vi "S4GUI_001.vi"() -> ()   [LabVIEW 2018] (continued)
            n2478 = call-dynamic "Read State Machine.vi"("error in (no error)"=w5934, "Device in"=w5935) -> ("error out"=w5938:errorcluster, "State Machine.lvclass"=w5931:refnum<class "State Machine.lvclass">, "Device out"=w5933:refnum<class "Channel.lvclass">)  [unwired: 7 in]
            n2479 = call "Next State.vi"("error in (no error)"=w5938, "New_State"=12, "State Machine in"=w5931) -> ("error out"=w5937:errorcluster, "State Machine out"=w5930:refnum<class "State Machine.lvclass">)  [unwired: 7 in]
            n2480 = call-dynamic "Write State Machine.vi"("error in (no error)"=w5937, "State Machine.lvclass"=w5930, "Device in"=w5933) -> ("error out"=w5929:errorcluster, "Device out"=w5932:refnum<class "Channel.lvclass">)  [unwired: 7 in]
            n2481 = call-dynamic "Write Channel.vi"("error in (no error)"=w5929, "Channel.lvclass"=w5932, "Acquisition in"=w5951) -> ("error out"=w5949:errorcluster, "Acquisition out"=w5950:refnum<class "Acquisition.lvclass">)  [unwired: 7 in]
            n2482 = call-dynamic "Write AcquisitionC.vi"("error in (no error)"=w5949, "Acquisition.lvclass"=w5950, "S4ACS_GUI in"=w5952) -> ("error out"=w5963:errorcluster, "S4ACS_GUI out"=w5964:refnum<class "S4GUI.lvclass">)  [unwired: 7 in]
          }
          frame #3 {
            # "object"
            # "suffix"
            # "obsType"
            n2483 = call-dynamic "Read AcquisitionD.vi"("error in (no error)"=w6008, "S4ACS_GUI in"=w6009) -> ("error out"=w6001:errorcluster, "Acquisition.lvclass"=w6000:refnum<class "Acquisition.lvclass">, "S4ACS_GUI out"=w5995:refnum<class "S4GUI.lvclass">)  [unwired: 7 in]
            n2484 = call-dynamic "Read Channel.vi"("error in (no error)"=w6001, "Acquisition in"=w6000) -> ("error out"=w5968:errorcluster, "Channel.lvclass"=w5970:refnum<class "Channel.lvclass">, "Acquisition out"=w5994:refnum<class "Acquisition.lvclass">)  [unwired: 7 in]
            n2485 = local read "Filter4"() -> (w5971:u8)
            n2486 = call-dynamic "Write Filter.vi"("error in (no error)"=w5968, "Filter"=w5971, "Channel in"=w5970) -> ("error out"=w5967:errorcluster, "Channel out"=w5969:refnum<class "Channel.lvclass">)  [unwired: 7 in]
            n2487 = call-dynamic "Read Interface.vi"("error in (no error)"=w5967, "Channel in"=w5969) -> ("error out"=w5986:errorcluster, "Interface.lvclass"=w5987:refnum<class "Interface.lvclass">, "Channel out"=w5999:refnum<class "Channel.lvclass">)  [unwired: 7 in]
            n2488 = call-dynamic "Write Suffix.vi"("error in (no error)"=w5986, "Suffix"=w6005, "Interface in"=w5987) -> ("error out"=w6004:errorcluster, "Interface out"=w5998:refnum<class "Interface.lvclass">)  [unwired: 7 in]
            n2489 = call-dynamic "Write ObsType.vi"("error in (no error)"=w6004, "ObsType"=w5990, "Interface in"=w5998) -> ("error out"=w6003:errorcluster, "Interface out"=w5997:refnum<class "Interface.lvclass">)  [unwired: 7 in]
            n2490 = call-dynamic "Write Object.vi"("error in (no error)"=w6003, "Object"=w5989, "Interface in"=w5997) -> ("error out"=w6002:errorcluster, "Interface out"=w5996:refnum<class "Interface.lvclass">)  [unwired: 7 in]
            n2491 = call-dynamic "Write Comments.vi"("error in (no error)"=w6002, "Comments"=w5991, "Interface in"=w5996) -> ("error out"=w5985:errorcluster, "Interface out"=w5984:refnum<class "Interface.lvclass">)  [unwired: 7 in]
            n2492 = call-dynamic "Write Observer.vi"("error in (no error)"=w5985, "Observer"=w5988, "Interface in"=w5984) -> ("error out"=w5980:errorcluster, "Interface out"=w5979:refnum<class "Interface.lvclass">)  [unwired: 7 in]
            n2493 = call-dynamic "Write Interface.vi"("error in (no error)"=w5980, "Interface.lvclass"=w5979, "Channel in"=w5999) -> ("error out"=w5975:errorcluster, "Channel out"=w5978:refnum<class "Channel.lvclass">)  [unwired: 7 in]
            n2494 = call-dynamic "Read State Machine.vi"("error in (no error)"=w5975, "Device in"=w5978) -> ("error out"=w5983:errorcluster, "State Machine.lvclass"=w5973:refnum<class "State Machine.lvclass">, "Device out"=w5977:refnum<class "Channel.lvclass">)  [unwired: 7 in]
            n2495 = call "Next State.vi"("error in (no error)"=w5983, "New_State"=12, "State Machine in"=w5973) -> ("error out"=w5982:errorcluster, "State Machine out"=w5972:refnum<class "State Machine.lvclass">)  [unwired: 7 in]
            n2496 = call-dynamic "Write State Machine.vi"("error in (no error)"=w5982, "State Machine.lvclass"=w5972, "Device in"=w5977) -> ("error out"=w5974:errorcluster, "Device out"=w5976:refnum<class "Channel.lvclass">)  [unwired: 7 in]
            n2497 = call-dynamic "Write Channel.vi"("error in (no error)"=w5974, "Channel.lvclass"=w5976, "Acquisition in"=w5994) -> ("error out"=w5992:errorcluster, "Acquisition out"=w5993:refnum<class "Acquisition.lvclass">)  [unwired: 7 in]
            n2498 = call-dynamic "Write AcquisitionD.vi"("error in (no error)"=w5992, "Acquisition.lvclass"=w5993, "S4ACS_GUI in"=w5995) -> ("error out"=w6006:errorcluster, "S4ACS_GUI out"=w6007:refnum<class "S4GUI.lvclass">)  [unwired: 7 in]
          }
        }
      }
      event "Start ch1": Value Change {
        n2499 = event-data() -> ()  [unwired: 1 in, 6 out]
        n2500 = call "Read Instrument.lvclass.vi"("error in (no error)"=w6016, "S4ACS_GUI in"=w6018) -> ("error out"=w6019:errorcluster, "Instrument.lvclass"=w6020:refnum<class "Instrument.lvclass">, "S4ACS_GUI out"=w6017:refnum<class "S4GUI.lvclass">)  [unwired: 7 in]
        n2501 = call-dynamic "Read mode.vi"("error in (no error)"=w6019, "Instrument in"=w6020) -> ("error out"=w6015:errorcluster, "mode"=w6014:bool)  [unwired: 7 in, 1 out]
        n2502 = call-dynamic "Read AcquisitionA.vi"("error in (no error)"=w6015, "S4ACS_GUI in"=w6017) -> ("error out"=w6032:errorcluster, "Acquisition.lvclass"=w6033:refnum<class "Acquisition.lvclass">, "S4ACS_GUI out"=w6035:refnum<class "S4GUI.lvclass">)  [unwired: 7 in]
        n2503 = call-dynamic "Read Acq_state.vi"("error in (no error)"=w6032, "Acquisition in"=w6033) -> ("error out"=w6029:errorcluster, "Acq_state"=w6031:u32, "Acquisition out"=w6028:refnum<class "Acquisition.lvclass">)  [unwired: 7 in]
        n2504 = Not Equal?(x=w6031, y=u32 400) -> (x != y?=w6034:bool)
        n2505 = case shown="True" w6034 {
          tunnel: w6035 -> [w6048 w6075]
          tunnel: [w6048 w6083] -> w6027
          tunnel: [w6036 w6081] -> w6011
          tunnel: w6029 -> [w6050 w6100]
          tunnel: w6028 -> [w6053 w6104]
          tunnel: [w6037 w6103] -> w6026
          tunnel: w6025 -> [_ w6102]
          tunnel: w6024 -> [_ w6101]
          tunnel: w6023 -> [_ w6099]
          tunnel: w6022 -> [_ w6098]
          tunnel: w6021 -> [_ w6093]
          tunnel: w6014 -> [_ w6080]
          tunnel: w6010 -> [_ w6066]
          frame False {
            n2506 = call-dynamic "Read Acq_prevstate.vi"("error in (no error)"=w6050, "Acquisition in"=w6053) -> ("error out"=w6049:errorcluster, "Acq_prevstate"=w6051:u32, "Acquisition out"=w6052:refnum<class "Acquisition.lvclass">)  [unwired: 7 in]
            n2507 = call-dynamic "Write Acq_state.vi"("error in (no error)"=w6049, "Acq_state"=w6051, "Acquisition in"=w6052) -> ("error out"=w6038:errorcluster, "Acquisition out"=w6039:refnum<class "Acquisition.lvclass">)  [unwired: 7 in]
            n2508 = call-dynamic "Read Channel.vi"("error in (no error)"=w6038, "Acquisition in"=w6039) -> ("error out"=w6042:errorcluster, "Channel.lvclass"=w6043:refnum<class "Channel.lvclass">, "Acquisition out"=w6047:refnum<class "Acquisition.lvclass">)  [unwired: 7 in]
            n2509 = call "Read connected.vi"("error in (no error)"=w6042, "Device in"=w6043) -> ("error out"=w6041:errorcluster, "connected"=w6040:bool, "Device out"=w6044:refnum<class "Channel.lvclass">)  [unwired: 7 in]
            n2510 = case shown="True" w6040 {
              tunnel: w6044 -> [w6055 w6065]
              tunnel: [w6055 w6063] -> w6046
              tunnel: w6041 -> [w6054 w6060]
              tunnel: [w6054 w6058] -> w6045
              frame False {
              }
              frame True {
                n2511 = call-dynamic "Read State Machine.vi"("error in (no error)"=w6060, "Device in"=w6065) -> ("error out"=w6056:errorcluster, "State Machine.lvclass"=w6057:refnum<class "State Machine.lvclass">, "Device out"=w6064:refnum<class "Channel.lvclass">)  [unwired: 7 in]
                n2512 = call "Next State.vi"("error in (no error)"=w6056, "New_State"=96, "State Machine in"=w6057) -> ("error out"=w6059:errorcluster, "State Machine out"=w6062:refnum<class "State Machine.lvclass">)  [unwired: 7 in]
                n2513 = call-dynamic "Write State Machine.vi"("error in (no error)"=w6059, "State Machine.lvclass"=w6062, "Device in"=w6064) -> ("error out"=w6058:errorcluster, "Device out"=w6063:refnum<class "Channel.lvclass">)  [unwired: 7 in]
              }
            }
            n2514 = call-dynamic "Write Channel.vi"("error in (no error)"=w6045, "Channel.lvclass"=w6046, "Acquisition in"=w6047) -> ("error out"=w6036:errorcluster, "Acquisition out"=w6037:refnum<class "Acquisition.lvclass">)  [unwired: 7 in]
          }
          frame True {
            # "object"
            # "suffix"
            # "obsType"
            n2515 = call "Read Instrument.lvclass.vi"("S4ACS_GUI in"=w6075) -> ("error out"=w6077:errorcluster, "Instrument.lvclass"=w6079:refnum<class "Instrument.lvclass">, "S4ACS_GUI out"=w6074:refnum<class "S4GUI.lvclass">)  [unwired: 8 in]
            n2516 = call "Read WPROT.vi"("error in (no error)"=w6077, "Instrument in"=w6079) -> ("error out"=w6076:errorcluster, "Opt_Selector.lvclass"=w6078:refnum<class "Opt_Selector.lvclass">)  [unwired: 7 in, 1 out]
            n2517 = call-dynamic "Read sequencia.vi"("error in (no error)"=w6076, "Opt_Selector in"=w6078) -> ("sequencia"=w6073:u16)  [unwired: 7 in, 2 out]
            n2518 = case shown="True" w6080 {
              tunnel: [0 w6141] -> w6072
              tunnel: w6073 -> [_ w6140]
              frame False {
                # "OV 20230424: \n#SEQ agora armazena as\nposições da lâmina utilizadas.\nNa fotometria, #SEQ=0"
                # "fotometria:"
              }
              frame True {
                # "OV 20230424: \n#SEQ agora armazena as\nposições da lâmina utilizadas.\nNa polarimetria, #SEQ=WPROT.sequencia"
                # "polarimetria:"
                n2519 = To Unsigned Long Integer(number=w6140) -> (unsigned 32bit integer=w6141:u32)
              }
            }
            n2520 = call-dynamic "Write Acq_state.vi"("error in (no error)"=w6100, "Acq_state"=u32 251, "Acquisition in"=w6104) -> ("error out"=w6105:errorcluster, "Acquisition out"=w6106:refnum<class "Acquisition.lvclass">)  [unwired: 7 in]
            n2521 = call-dynamic "Read Channel.vi"("error in (no error)"=w6105, "Acquisition in"=w6106) -> ("error out"=w6108:errorcluster, "Channel.lvclass"=w6109:refnum<class "Channel.lvclass">, "Acquisition out"=w6120:refnum<class "Acquisition.lvclass">)  [unwired: 7 in]
            n2522 = property on="Start ch1" class="Bool"(error in=w6100, "DisabledEnum"=T7."Disabled and Grayed Out" ("Disabled")) -> ()  [unwired: 1 in, 2 out]
            n2523 = call-dynamic "Read Interface.vi"("error in (no error)"=w6108, "Channel in"=w6109) -> ("error out"=w6130:errorcluster, "Interface.lvclass"=w6131:refnum<class "Interface.lvclass">, "Channel out"=w6129:refnum<class "Channel.lvclass">)  [unwired: 7 in]
            n2524 = call "Write Exposure Time.vi"("error in (no error)"=w6130, "Exposure Time"="Exptime ch1", "Interface in"=w6131) -> ("error out"=w6070:errorcluster, "Interface out"=w6071:refnum<class "Interface.lvclass">)  [unwired: 7 in]
            n2525 = case shown="\"ZERO\"" w6066 {
              tunnel: w6071 -> [w6133 w6138]
              tunnel: w6070 -> [w6132 w6137]
              tunnel: "Exptime ch1" -> [_ w6136]
              tunnel: [w6132 w6135] -> w6068
              tunnel: [w6133 w6134] -> w6067
              frame "ZERO" {
              }
              frame Default {
                n2526 = call-dynamic "Write prev ExpTime.vi"("error in (no error)"=w6137, "prev ExpTime"=w6136, "Interface in"=w6138) -> ("error out"=w6135:errorcluster, "Interface out"=w6134:refnum<class "Interface.lvclass">)  [unwired: 7 in]
              }
            }
            n2527 = call-dynamic "Write Suffix.vi"("error in (no error)"=w6068, "Suffix"=w6102, "Interface in"=w6067) -> ("error out"=w6128:errorcluster, "Interface out"=w6127:refnum<class "Interface.lvclass">)  [unwired: 7 in]
            n2528 = call-dynamic "Write ObsType.vi"("error in (no error)"=w6128, "ObsType"=w6099, "Interface in"=w6127) -> ("error out"=w6125:errorcluster, "Interface out"=w6126:refnum<class "Interface.lvclass">)  [unwired: 7 in]
            n2529 = call-dynamic "Write Object.vi"("error in (no error)"=w6125, "Object"=w6098, "Interface in"=w6126) -> ("error out"=w6124:errorcluster, "Interface out"=w6123:refnum<class "Interface.lvclass">)  [unwired: 7 in]
            n2530 = call-dynamic "Write Comments.vi"("error in (no error)"=w6124, "Comments"=w6101, "Interface in"=w6123) -> ("error out"=w6121:errorcluster, "Interface out"=w6122:refnum<class "Interface.lvclass">)  [unwired: 7 in]
            n2531 = call-dynamic "Write DS9.vi"("error in (no error)"=w6121, "DS9"="F", "Interface in"=w6122) -> ("error out"=w6095:errorcluster, "Interface out"=w6097:refnum<class "Interface.lvclass">)  [unwired: 7 in]
            n2532 = call-dynamic "Write Observer.vi"("error in (no error)"=w6095, "Observer"=w6093, "Interface in"=w6097) -> ("error out"=w6094:errorcluster, "Interface out"=w6096:refnum<class "Interface.lvclass">)  [unwired: 7 in]
            n2533 = call-dynamic "Write # Images.vi"("error in (no error)"=w6094, "# Images"="Exp ch1", "Interface in"=w6096) -> ("error out"=w6117:errorcluster, "Interface out"=w6119:refnum<class "Interface.lvclass">)  [unwired: 7 in]
            n2534 = call-dynamic "Write Interface.vi"("error in (no error)"=w6117, "Interface.lvclass"=w6119, "Channel in"=w6129) -> ("error out"=w6110:errorcluster, "Channel out"=w6111:refnum<class "Channel.lvclass">)  [unwired: 7 in]
            n2535 = property on="Exposure Time ch1" class="Slide (strict)"("Scale.Maximum"="Exptime ch1", "Scale.Minimum"=0.0 ("Scale.Range:Minimum")) -> ()  [unwired: 2 in, 2 out]
            n2536 = property on="Cycles Done ch1" class="Slide (strict)"("Scale.Maximum"="#cycles ch1", "Scale.Minimum"=0.0 ("Scale.Range:Minimum")) -> ()  [unwired: 2 in, 2 out]
            n2537 = property on="Exposure Done ch1" class="Slide (strict)"("Scale.Maximum"="Exp ch1", "Scale.Minimum"=0.0 ("Scale.Range:Minimum")) -> ()  [unwired: 2 in, 2 out]
            n2538 = call-dynamic "Write ciclos.vi"("error in (no error)"=w6110, "ciclos"="#cycles ch1", "Channel in"=w6111) -> ("error out"=w6091:errorcluster, "Channel out"=w6092:refnum<class "Channel.lvclass">)  [unwired: 7 in]
            n2539 = call-dynamic "Write sequencias.vi"("error in (no error)"=w6091, "sequencias"=w6072, "Channel in"=w6092) -> ("error out"=w6090:errorcluster, "Channel out"=w6089:refnum<class "Channel.lvclass">)  [unwired: 7 in]
            n2540 = call-dynamic "Write Channel.vi"("error in (no error)"=w6090, "Channel.lvclass"=w6089, "Acquisition in"=w6120) -> ("error out"=w6082:errorcluster, "Acquisition out"=w6103:refnum<class "Acquisition.lvclass">)  [unwired: 7 in]
            n2541 = call-dynamic "Write sequencias.vi"("error in (no error)"=w6082, "sequencias"=w6072, "S4GUI in"=w6074) -> ("error out"=w6086:errorcluster, "S4GUI out"=w6085:refnum<class "S4GUI.lvclass">)  [unwired: 7 in]
            n2542 = call-dynamic "Write ciclos.vi"("error in (no error)"=w6086, "ciclos"="#cycles ch1", "S4ACS_GUI in"=w6085) -> ("error out"=w6087:errorcluster, "S4ACS_GUI out"=w6088:refnum<class "S4GUI.lvclass">)  [unwired: 7 in]
            n2543 = call-dynamic "Write TotalCiclos.vi"("error in (no error)"=w6087, "TotalCiclos"="#cycles ch1", "S4GUI in"=w6088) -> ("error out"=w6081:errorcluster, "S4GUI out"=w6083:refnum<class "S4GUI.lvclass">)  [unwired: 7 in]
          }
        }
        n2544 = call-dynamic "Write AcquisitionA.vi"("error in (no error)"=w6011, "Acquisition.lvclass"=w6026, "S4ACS_GUI in"=w6027) -> ("error out"=w6012:errorcluster, "S4ACS_GUI out"=w6013:refnum<class "S4GUI.lvclass">)  [unwired: 7 in]
      }
      event "Start ch2": Value Change {
        n2545 = event-data() -> ()  [unwired: 1 in, 6 out]
        n2546 = call "Read Instrument.lvclass.vi"("error in (no error)"=w6146, "S4ACS_GUI in"=w6147) -> ("error out"=w6148:errorcluster, "Instrument.lvclass"=w6149:refnum<class "Instrument.lvclass">, "S4ACS_GUI out"=w6145:refnum<class "S4GUI.lvclass">)  [unwired: 7 in]
        n2547 = call-dynamic "Read mode.vi"("error in (no error)"=w6148, "Instrument in"=w6149) -> ("error out"=w6144:errorcluster, "mode"=w6143:bool)  [unwired: 7 in, 1 out]
        n2548 = call "Read AcquisitionB.vi"("error in (no error)"=w6144, "S4ACS_GUI in"=w6145) -> ("error out"=w6163:errorcluster, "Acquisition.lvclass"=w6164:refnum<class "Acquisition.lvclass">, "S4ACS_GUI out"=w6166:refnum<class "S4GUI.lvclass">)  [unwired: 7 in]
        n2549 = call-dynamic "Read Acq_state.vi"("error in (no error)"=w6163, "Acquisition in"=w6164) -> ("error out"=w6160:errorcluster, "Acq_state"=w6162:u32, "Acquisition out"=w6159:refnum<class "Acquisition.lvclass">)  [unwired: 7 in]
        n2550 = Not Equal?(x=w6162, y=u32 400) -> (x != y?=w6165:bool)
        n2551 = case shown="True" w6165 {
          tunnel: w6166 -> [w6179 w6206]
          tunnel: [w6179 w6214] -> w6158
          tunnel: [w6167 w6212] -> w6142
          tunnel: w6160 -> [w6181 w6234]
          tunnel: w6159 -> [w6184 w6239]
          tunnel: [w6168 w6238] -> w6157
          tunnel: w6155 -> [_ w6236]
          tunnel: w6154 -> [_ w6235]
          tunnel: w6152 -> [_ w6230]
          tunnel: w6151 -> [_ w6229]
          tunnel: w6150 -> [_ w6223]
          tunnel: w6143 -> [_ w6203]
          frame False {
            n2552 = call-dynamic "Read Acq_prevstate.vi"("error in (no error)"=w6181, "Acquisition in"=w6184) -> ("error out"=w6180:errorcluster, "Acq_prevstate"=w6182:u32, "Acquisition out"=w6183:refnum<class "Acquisition.lvclass">)  [unwired: 7 in]
            n2553 = call-dynamic "Write Acq_state.vi"("error in (no error)"=w6180, "Acq_state"=w6182, "Acquisition in"=w6183) -> ("error out"=w6169:errorcluster, "Acquisition out"=w6170:refnum<class "Acquisition.lvclass">)  [unwired: 7 in]
            n2554 = call-dynamic "Read Channel.vi"("error in (no error)"=w6169, "Acquisition in"=w6170) -> ("error out"=w6173:errorcluster, "Channel.lvclass"=w6174:refnum<class "Channel.lvclass">, "Acquisition out"=w6178:refnum<class "Acquisition.lvclass">)  [unwired: 7 in]
            n2555 = call "Read connected.vi"("error in (no error)"=w6173, "Device in"=w6174) -> ("error out"=w6172:errorcluster, "connected"=w6171:bool, "Device out"=w6175:refnum<class "Channel.lvclass">)  [unwired: 7 in]
            n2556 = case shown="True" w6171 {
              tunnel: w6175 -> [w6186 w6196]
              tunnel: [w6186 w6194] -> w6177
              tunnel: w6172 -> [w6185 w6191]
              tunnel: [w6185 w6189] -> w6176
              frame False {
              }
              frame True {
                n2557 = call-dynamic "Read State Machine.vi"("error in (no error)"=w6191, "Device in"=w6196) -> ("error out"=w6187:errorcluster, "State Machine.lvclass"=w6188:refnum<class "State Machine.lvclass">, "Device out"=w6195:refnum<class "Channel.lvclass">)  [unwired: 7 in]
                n2558 = call "Next State.vi"("error in (no error)"=w6187, "New_State"=96, "State Machine in"=w6188) -> ("error out"=w6190:errorcluster, "State Machine out"=w6193:refnum<class "State Machine.lvclass">)  [unwired: 7 in]
                n2559 = call-dynamic "Write State Machine.vi"("error in (no error)"=w6190, "State Machine.lvclass"=w6193, "Device in"=w6195) -> ("error out"=w6189:errorcluster, "Device out"=w6194:refnum<class "Channel.lvclass">)  [unwired: 7 in]
              }
            }
            n2560 = call-dynamic "Write Channel.vi"("error in (no error)"=w6176, "Channel.lvclass"=w6177, "Acquisition in"=w6178) -> ("error out"=w6167:errorcluster, "Acquisition out"=w6168:refnum<class "Acquisition.lvclass">)  [unwired: 7 in]
          }
          frame True {
            # "obs type"
            # "suffix"
            # "object"
            n2561 = call "Read Instrument.lvclass.vi"("S4ACS_GUI in"=w6206) -> ("error out"=w6208:errorcluster, "Instrument.lvclass"=w6210:refnum<class "Instrument.lvclass">, "S4ACS_GUI out"=w6205:refnum<class "S4GUI.lvclass">)  [unwired: 8 in]
            n2562 = call "Read WPROT.vi"("error in (no error)"=w6208, "Instrument in"=w6210) -> ("error out"=w6207:errorcluster, "Opt_Selector.lvclass"=w6209:refnum<class "Opt_Selector.lvclass">)  [unwired: 7 in, 1 out]
            n2563 = call-dynamic "Read sequencia.vi"("error in (no error)"=w6207, "Opt_Selector in"=w6209) -> ("sequencia"=w6202:u16)  [unwired: 7 in, 2 out]
            n2564 = case shown="True" w6203 {
              tunnel: [0 w6267] -> w6204
              tunnel: w6202 -> [_ w6266]
              frame False {
                # "OV 20230424: \n#SEQ agora armazena as\nposições da lâmina utilizadas.\nNa fotometria, #SEQ=0"
                # "fotometria:"
              }
              frame True {
                # "OV 20230424: \n#SEQ agora armazena as\nposições da lâmina utilizadas.\nNa polarimetria, #SEQ=WPROT.sequencia"
                # "polarimetria:"
                n2565 = To Unsigned Long Integer(number=w6266) -> (unsigned 32bit integer=w6267:u32)
              }
            }
            n2566 = call-dynamic "Write Acq_state.vi"("error in (no error)"=w6234, "Acq_state"=u32 251, "Acquisition in"=w6239) -> ("error out"=w6240:errorcluster, "Acquisition out"=w6241:refnum<class "Acquisition.lvclass">)  [unwired: 7 in]
            n2567 = call-dynamic "Read Channel.vi"("error in (no error)"=w6240, "Acquisition in"=w6241) -> ("error out"=w6243:errorcluster, "Channel.lvclass"=w6244:refnum<class "Channel.lvclass">, "Acquisition out"=w6251:refnum<class "Acquisition.lvclass">)  [unwired: 7 in]
            n2568 = property on="Start ch2" class="Bool"(error in=w6234, "DisabledEnum"=T7."Disabled and Grayed Out" ("Disabled")) -> ()  [unwired: 1 in, 2 out]
            n2569 = call-dynamic "Read Interface.vi"("error in (no error)"=w6243, "Channel in"=w6244) -> ("error out"=w6263:errorcluster, "Interface.lvclass"=w6264:refnum<class "Interface.lvclass">, "Channel out"=w6262:refnum<class "Channel.lvclass">)  [unwired: 7 in]
            n2570 = call "Write Exposure Time.vi"("error in (no error)"=w6263, "Exposure Time"="Exptime ch2", "Interface in"=w6264) -> ("error out"=w6199:errorcluster, "Interface out"=w6201:refnum<class "Interface.lvclass">)  [unwired: 7 in]
            n2571 = call-dynamic "Write prev ExpTime.vi"("error in (no error)"=w6199, "prev ExpTime"="Exptime ch2", "Interface in"=w6201) -> ("error out"=w6198:errorcluster, "Interface out"=w6200:refnum<class "Interface.lvclass">)  [unwired: 7 in]
            n2572 = call-dynamic "Write # Index.vi"("error in (no error)"=w6198, "# Index"="Index ch2", "Interface in"=w6200) -> ("error out"=w6260:errorcluster, "Interface out"=w6261:refnum<class "Interface.lvclass">)  [unwired: 7 in]
            n2573 = call-dynamic "Write Suffix.vi"("error in (no error)"=w6260, "Suffix"=w6236, "Interface in"=w6261) -> ("error out"=w6259:errorcluster, "Interface out"=w6258:refnum<class "Interface.lvclass">)  [unwired: 7 in]
            n2574 = call-dynamic "Write ObsType.vi"("error in (no error)"=w6259, "ObsType"=w6230, "Interface in"=w6258) -> ("error out"=w6256:errorcluster, "Interface out"=w6257:refnum<class "Interface.lvclass">)  [unwired: 7 in]
            n2575 = call-dynamic "Write Object.vi"("error in (no error)"=w6256, "Object"=w6229, "Interface in"=w6257) -> ("error out"=w6255:errorcluster, "Interface out"=w6254:refnum<class "Interface.lvclass">)  [unwired: 7 in]
            n2576 = call-dynamic "Write Comments.vi"("error in (no error)"=w6255, "Comments"=w6235, "Interface in"=w6254) -> ("error out"=w6252:errorcluster, "Interface out"=w6253:refnum<class "Interface.lvclass">)  [unwired: 7 in]
            n2577 = call-dynamic "Write DS9.vi"("error in (no error)"=w6252, "DS9"="F", "Interface in"=w6253) -> ("error out"=w6226:errorcluster, "Interface out"=w6228:refnum<class "Interface.lvclass">)  [unwired: 7 in]
            n2578 = call-dynamic "Write Observer.vi"("error in (no error)"=w6226, "Observer"=w6223, "Interface in"=w6228) -> ("error out"=w6225:errorcluster, "Interface out"=w6227:refnum<class "Interface.lvclass">)  [unwired: 7 in]
            n2579 = call-dynamic "Write # Images.vi"("error in (no error)"=w6225, "# Images"="Exp ch2", "Interface in"=w6227) -> ("error out"=w6232:errorcluster, "Interface out"=w6231:refnum<class "Interface.lvclass">)  [unwired: 7 in]
            n2580 = property on="Exposure Time ch2" class="Slide (strict)"("Scale.Maximum"="Exptime ch2", "Scale.Minimum"=0.0 ("Scale.Range:Minimum")) -> ()  [unwired: 2 in, 2 out]
            n2581 = property on="Cycles Done ch2" class="Slide (strict)"("Scale.Maximum"="#cycles ch2", "Scale.Minimum"=0.0 ("Scale.Range:Minimum")) -> ()  [unwired: 2 in, 2 out]
            n2582 = property on="Exposure Done ch2" class="Slide (strict)"("Scale.Maximum"="Exp ch2", "Scale.Minimum"=0.0 ("Scale.Range:Minimum")) -> ()  [unwired: 2 in, 2 out]
            n2583 = call-dynamic "Write Interface.vi"("error in (no error)"=w6232, "Interface.lvclass"=w6231, "Channel in"=w6262) -> ("error out"=w6245:errorcluster, "Channel out"=w6246:refnum<class "Channel.lvclass">)  [unwired: 7 in]
            n2584 = call-dynamic "Write ciclos.vi"("error in (no error)"=w6245, "ciclos"="#cycles ch2", "Channel in"=w6246) -> ("error out"=w6222:errorcluster, "Channel out"=w6221:refnum<class "Channel.lvclass">)  [unwired: 7 in]
            n2585 = call-dynamic "Write sequencias.vi"("error in (no error)"=w6222, "sequencias"=w6204, "Channel in"=w6221) -> ("error out"=w6220:errorcluster, "Channel out"=w6219:refnum<class "Channel.lvclass">)  [unwired: 7 in]
            n2586 = call-dynamic "Write Channel.vi"("error in (no error)"=w6220, "Channel.lvclass"=w6219, "Acquisition in"=w6251) -> ("error out"=w6213:errorcluster, "Acquisition out"=w6238:refnum<class "Acquisition.lvclass">)  [unwired: 7 in]
            n2587 = call-dynamic "Write sequencias.vi"("error in (no error)"=w6213, "sequencias"=w6204, "S4GUI in"=w6205) -> ("error out"=w6216:errorcluster, "S4GUI out"=w6215:refnum<class "S4GUI.lvclass">)  [unwired: 7 in]
            n2588 = call-dynamic "Write ciclos.vi"("error in (no error)"=w6216, "ciclos"="#cycles ch2", "S4ACS_GUI in"=w6215) -> ("error out"=w6217:errorcluster, "S4ACS_GUI out"=w6218:refnum<class "S4GUI.lvclass">)  [unwired: 7 in]
            n2589 = call-dynamic "Write TotalCiclos.vi"("error in (no error)"=w6217, "TotalCiclos"="#cycles ch2", "S4GUI in"=w6218) -> ("error out"=w6212:errorcluster, "S4GUI out"=w6214:refnum<class "S4GUI.lvclass">)  [unwired: 7 in]
          }
        }
        n2590 = call "Write AcquisitionB.vi"("error in (no error)"=w6142, "Acquisition.lvclass"=w6157, "S4ACS_GUI in"=w6158) -> ("error out"=w6156:errorcluster, "S4ACS_GUI out"=w6153:refnum<class "S4GUI.lvclass">)  [unwired: 7 in]
      }
      event "Start ch3": Value Change {
        n2591 = event-data() -> ()  [unwired: 1 in, 6 out]
        n2592 = call "Read Instrument.lvclass.vi"("error in (no error)"=w6271, "S4ACS_GUI in"=w6273) -> ("error out"=w6274:errorcluster, "Instrument.lvclass"=w6275:refnum<class "Instrument.lvclass">, "S4ACS_GUI out"=w6272:refnum<class "S4GUI.lvclass">)  [unwired: 7 in]
        n2593 = call-dynamic "Read mode.vi"("error in (no error)"=w6274, "Instrument in"=w6275) -> ("error out"=w6270:errorcluster, "mode"=w6269:bool)  [unwired: 7 in, 1 out]
        n2594 = call-dynamic "Read AcquisitionC.vi"("error in (no error)"=w6270, "S4ACS_GUI in"=w6272) -> ("error out"=w6289:errorcluster, "Acquisition.lvclass"=w6290:refnum<class "Acquisition.lvclass">, "S4ACS_GUI out"=w6292:refnum<class "S4GUI.lvclass">)  [unwired: 7 in]
        n2595 = call-dynamic "Read Acq_state.vi"("error in (no error)"=w6289, "Acquisition in"=w6290) -> ("error out"=w6286:errorcluster, "Acq_state"=w6288:u32, "Acquisition out"=w6285:refnum<class "Acquisition.lvclass">)  [unwired: 7 in]
        n2596 = Not Equal?(x=w6288, y=u32 400) -> (x != y?=w6291:bool)
        n2597 = case shown="True" w6291 {
          tunnel: w6292 -> [w6305 w6330]
          tunnel: [w6305 w6338] -> w6284
          tunnel: [w6293 w6339] -> w6268
          tunnel: w6286 -> [w6307 w6359]
          tunnel: w6285 -> [w6310 w6364]
          tunnel: [w6294 w6363] -> w6283
          tunnel: w6281 -> [_ w6361]
          tunnel: w6280 -> [_ w6360]
          tunnel: w6278 -> [_ w6355]
          tunnel: w6277 -> [_ w6354]
          tunnel: w6276 -> [_ w6349]
          tunnel: w6269 -> [_ w6335]
          frame False {
            n2598 = call-dynamic "Read Acq_prevstate.vi"("error in (no error)"=w6307, "Acquisition in"=w6310) -> ("error out"=w6306:errorcluster, "Acq_prevstate"=w6308:u32, "Acquisition out"=w6309:refnum<class "Acquisition.lvclass">)  [unwired: 7 in]
            n2599 = call-dynamic "Write Acq_state.vi"("error in (no error)"=w6306, "Acq_state"=w6308, "Acquisition in"=w6309) -> ("error out"=w6298:errorcluster, "Acquisition out"=w6299:refnum<class "Acquisition.lvclass">)  [unwired: 7 in]
            n2600 = call-dynamic "Read Channel.vi"("error in (no error)"=w6298, "Acquisition in"=w6299) -> ("error out"=w6302:errorcluster, "Channel.lvclass"=w6296:refnum<class "Channel.lvclass">, "Acquisition out"=w6297:refnum<class "Acquisition.lvclass">)  [unwired: 7 in]
            n2601 = call "Read connected.vi"("error in (no error)"=w6302, "Device in"=w6296) -> ("error out"=w6301:errorcluster, "connected"=w6300:bool, "Device out"=w6303:refnum<class "Channel.lvclass">)  [unwired: 7 in]
            n2602 = case shown="True" w6300 {
              tunnel: w6303 -> [w6312 w6322]
              tunnel: [w6312 w6320] -> w6295
              tunnel: w6301 -> [w6311 w6317]
              tunnel: [w6311 w6315] -> w6304
              frame False {
              }
              frame True {
                n2603 = call-dynamic "Read State Machine.vi"("error in (no error)"=w6317, "Device in"=w6322) -> ("error out"=w6313:errorcluster, "State Machine.lvclass"=w6314:refnum<class "State Machine.lvclass">, "Device out"=w6321:refnum<class "Channel.lvclass">)  [unwired: 7 in]
                n2604 = call "Next State.vi"("error in (no error)"=w6313, "New_State"=96, "State Machine in"=w6314) -> ("error out"=w6316:errorcluster, "State Machine out"=w6319:refnum<class "State Machine.lvclass">)  [unwired: 7 in]
                n2605 = call-dynamic "Write State Machine.vi"("error in (no error)"=w6316, "State Machine.lvclass"=w6319, "Device in"=w6321) -> ("error out"=w6315:errorcluster, "Device out"=w6320:refnum<class "Channel.lvclass">)  [unwired: 7 in]
              }
            }
            n2606 = call-dynamic "Write Channel.vi"("error in (no error)"=w6304, "Channel.lvclass"=w6295, "Acquisition in"=w6297) -> ("error out"=w6293:errorcluster, "Acquisition out"=w6294:refnum<class "Acquisition.lvclass">)  [unwired: 7 in]
          }
          frame True {
            # "obs type"
            # "suffix"
            # "object"
            n2607 = call "Read Instrument.lvclass.vi"("S4ACS_GUI in"=w6330) -> ("error out"=w6332:errorcluster, "Instrument.lvclass"=w6334:refnum<class "Instrument.lvclass">, "S4ACS_GUI out"=w6329:refnum<class "S4GUI.lvclass">)  [unwired: 8 in]
            n2608 = call "Read WPROT.vi"("error in (no error)"=w6332, "Instrument in"=w6334) -> ("error out"=w6331:errorcluster, "Opt_Selector.lvclass"=w6333:refnum<class "Opt_Selector.lvclass">)  [unwired: 7 in, 1 out]
            n2609 = call-dynamic "Read sequencia.vi"("error in (no error)"=w6331, "Opt_Selector in"=w6333) -> ("sequencia"=w6328:u16)  [unwired: 7 in, 2 out]
            n2610 = case shown="True" w6335 {
              tunnel: [0 w6393] -> w6336
              tunnel: w6328 -> [_ w6392]
              frame False {
                # "OV 20230424: \n#SEQ agora armazena as\nposições da lâmina utilizadas.\nNa fotometria, #SEQ=0"
                # "fotometria:"
              }
              frame True {
                # "OV 20230424: \n#SEQ agora armazena as\nposições da lâmina utilizadas.\nNa polarimetria, #SEQ=WPROT.sequencia"
                # "polarimetria:"
                n2611 = To Unsigned Long Integer(number=w6392) -> (unsigned 32bit integer=w6393:u32)
              }
            }
            n2612 = call-dynamic "Write Acq_state.vi"("error in (no error)"=w6359, "Acq_state"=u32 251, "Acquisition in"=w6364) -> ("error out"=w6365:errorcluster, "Acquisition out"=w6366:refnum<class "Acquisition.lvclass">)  [unwired: 7 in]
            n2613 = call-dynamic "Read Channel.vi"("error in (no error)"=w6365, "Acquisition in"=w6366) -> ("error out"=w6368:errorcluster, "Channel.lvclass"=w6369:refnum<class "Channel.lvclass">, "Acquisition out"=w6377:refnum<class "Acquisition.lvclass">)  [unwired: 7 in]
            n2614 = property on="Start ch3" class="Bool"(error in=w6359, "DisabledEnum"=T7."Disabled and Grayed Out" ("Disabled")) -> ()  [unwired: 1 in, 2 out]
            n2615 = call-dynamic "Read Interface.vi"("error in (no error)"=w6368, "Channel in"=w6369) -> ("error out"=w6389:errorcluster, "Interface.lvclass"=w6390:refnum<class "Interface.lvclass">, "Channel out"=w6388:refnum<class "Channel.lvclass">)  [unwired: 7 in]
            n2616 = call "Write Exposure Time.vi"("error in (no error)"=w6389, "Exposure Time"="Exptime ch3", "Interface in"=w6390) -> ("error out"=w6325:errorcluster, "Interface out"=w6326:refnum<class "Interface.lvclass">)  [unwired: 7 in]
            n2617 = call-dynamic "Write prev ExpTime.vi"("error in (no error)"=w6325, "prev ExpTime"="Exptime ch3", "Interface in"=w6326) -> ("error out"=w6324:errorcluster, "Interface out"=w6327:refnum<class "Interface.lvclass">)  [unwired: 7 in]
            n2618 = call-dynamic "Write # Index.vi"("error in (no error)"=w6324, "# Index"="Index ch3", "Interface in"=w6327) -> ("error out"=w6386:errorcluster, "Interface out"=w6387:refnum<class "Interface.lvclass">)  [unwired: 7 in]
            n2619 = call-dynamic "Write Suffix.vi"("error in (no error)"=w6386, "Suffix"=w6361, "Interface in"=w6387) -> ("error out"=w6385:errorcluster, "Interface out"=w6384:refnum<class "Interface.lvclass">)  [unwired: 7 in]
            n2620 = call-dynamic "Write ObsType.vi"("error in (no error)"=w6385, "ObsType"=w6354, "Interface in"=w6384) -> ("error out"=w6382:errorcluster, "Interface out"=w6383:refnum<class "Interface.lvclass">)  [unwired: 7 in]
            n2621 = call-dynamic "Write Object.vi"("error in (no error)"=w6382, "Object"=w6355, "Interface in"=w6383) -> ("error out"=w6381:errorcluster, "Interface out"=w6380:refnum<class "Interface.lvclass">)  [unwired: 7 in]
            n2622 = call-dynamic "Write Comments.vi"("error in (no error)"=w6381, "Comments"=w6360, "Interface in"=w6380) -> ("error out"=w6378:errorcluster, "Interface out"=w6379:refnum<class "Interface.lvclass">)  [unwired: 7 in]
            n2623 = call-dynamic "Write DS9.vi"("error in (no error)"=w6378, "DS9"="F", "Interface in"=w6379) -> ("error out"=w6351:errorcluster, "Interface out"=w6353:refnum<class "Interface.lvclass">)  [unwired: 7 in]
            n2624 = call-dynamic "Write Observer.vi"("error in (no error)"=w6351, "Observer"=w6349, "Interface in"=w6353) -> ("error out"=w6350:errorcluster, "Interface out"=w6352:refnum<class "Interface.lvclass">)  [unwired: 7 in]
            n2625 = call-dynamic "Write # Images.vi"("error in (no error)"=w6350, "# Images"="Exp ch3", "Interface in"=w6352) -> ("error out"=w6356:errorcluster, "Interface out"=w6357:refnum<class "Interface.lvclass">)  [unwired: 7 in]
            n2626 = property on="Exposure Time ch3" class="Slide (strict)"("Scale.Maximum"="Exptime ch3", "Scale.Minimum"=0.0 ("Scale.Range:Minimum")) -> ()  [unwired: 2 in, 2 out]
            n2627 = property on="Exposure Done ch3" class="Slide (strict)"("Scale.Maximum"="Exp ch3", "Scale.Minimum"=0.0 ("Scale.Range:Minimum")) -> ()  [unwired: 2 in, 2 out]
            n2628 = property on="Cycles Done ch3" class="Slide (strict)"("Scale.Maximum"="#cycles ch3", "Scale.Minimum"=0.0 ("Scale.Range:Minimum")) -> ()  [unwired: 2 in, 2 out]
            n2629 = call-dynamic "Write Interface.vi"("error in (no error)"=w6356, "Interface.lvclass"=w6357, "Channel in"=w6388) -> ("error out"=w6370:errorcluster, "Channel out"=w6371:refnum<class "Channel.lvclass">)  [unwired: 7 in]
            n2630 = call-dynamic "Write ciclos.vi"("error in (no error)"=w6370, "ciclos"="#cycles ch3", "Channel in"=w6371) -> ("error out"=w6347:errorcluster, "Channel out"=w6348:refnum<class "Channel.lvclass">)  [unwired: 7 in]
            n2631 = call-dynamic "Write sequencias.vi"("error in (no error)"=w6347, "sequencias"=w6336, "Channel in"=w6348) -> ("error out"=w6345:errorcluster, "Channel out"=w6346:refnum<class "Channel.lvclass">)  [unwired: 7 in]
            n2632 = call-dynamic "Write Channel.vi"("error in (no error)"=w6345, "Channel.lvclass"=w6346, "Acquisition in"=w6377) -> ("error out"=w6340:errorcluster, "Acquisition out"=w6363:refnum<class "Acquisition.lvclass">)  [unwired: 7 in]
            n2633 = call-dynamic "Write sequencias.vi"("error in (no error)"=w6340, "sequencias"=w6336, "S4GUI in"=w6329) -> ("error out"=w6342:errorcluster, "S4GUI out"=w6341:refnum<class "S4GUI.lvclass">)  [unwired: 7 in]
            n2634 = call-dynamic "Write ciclos.vi"("error in (no error)"=w6342, "ciclos"="#cycles ch3", "S4ACS_GUI in"=w6341) -> ("error out"=w6343:errorcluster, "S4ACS_GUI out"=w6344:refnum<class "S4GUI.lvclass">)  [unwired: 7 in]
            n2635 = call-dynamic "Write TotalCiclos.vi"("error in (no error)"=w6343, "TotalCiclos"="#cycles ch3", "S4GUI in"=w6344) -> ("error out"=w6339:errorcluster, "S4GUI out"=w6338:refnum<class "S4GUI.lvclass">)  [unwired: 7 in]
          }
        }
        n2636 = call-dynamic "Write AcquisitionC.vi"("error in (no error)"=w6268, "Acquisition.lvclass"=w6283, "S4ACS_GUI in"=w6284) -> ("error out"=w6282:errorcluster, "S4ACS_GUI out"=w6279:refnum<class "S4GUI.lvclass">)  [unwired: 7 in]
      }
      event "Start ch4": Value Change {
        n2637 = event-data() -> ()  [unwired: 1 in, 6 out]
        n2638 = call "Read Instrument.lvclass.vi"("error in (no error)"=w6399, "S4ACS_GUI in"=w6400) -> ("error out"=w6401:errorcluster, "Instrument.lvclass"=w6402:refnum<class "Instrument.lvclass">, "S4ACS_GUI out"=w6398:refnum<class "S4GUI.lvclass">)  [unwired: 7 in]
        n2639 = call-dynamic "Read mode.vi"("error in (no error)"=w6401, "Instrument in"=w6402) -> ("error out"=w6397:errorcluster, "mode"=w6396:bool)  [unwired: 7 in, 1 out]
        n2640 = call-dynamic "Read AcquisitionD.vi"("error in (no error)"=w6397, "S4ACS_GUI in"=w6398) -> ("error out"=w6415:errorcluster, "Acquisition.lvclass"=w6416:refnum<class "Acquisition.lvclass">, "S4ACS_GUI out"=w6418:refnum<class "S4GUI.lvclass">)  [unwired: 7 in]
        n2641 = call-dynamic "Read Acq_state.vi"("error in (no error)"=w6415, "Acquisition in"=w6416) -> ("error out"=w6412:errorcluster, "Acq_state"=w6414:u32, "Acquisition out"=w6411:refnum<class "Acquisition.lvclass">)  [unwired: 7 in]
        n2642 = Not Equal?(x=w6414, y=u32 400) -> (x != y?=w6417:bool)
        n2643 = case shown="True" w6417 {
          tunnel: w6418 -> [w6431 w6456]
          tunnel: [w6420 w6464] -> w6395
          tunnel: w6412 -> [w6433 w6485]
          tunnel: w6411 -> [w6436 w6490]
          tunnel: [w6419 w6489] -> w6410
          tunnel: w6408 -> [_ w6487]
          tunnel: w6407 -> [_ w6486]
          tunnel: w6405 -> [_ w6481]
          tunnel: w6404 -> [_ w6480]
          tunnel: w6403 -> [_ w6475]
          tunnel: w6396 -> [_ w6462]
          tunnel: [w6431 w6466] -> w6394
          frame False {
            n2644 = call-dynamic "Read Acq_prevstate.vi"("error in (no error)"=w6433, "Acquisition in"=w6436) -> ("error out"=w6432:errorcluster, "Acq_prevstate"=w6434:u32, "Acquisition out"=w6435:refnum<class "Acquisition.lvclass">)  [unwired: 7 in]
            n2645 = call-dynamic "Write Acq_state.vi"("error in (no error)"=w6432, "Acq_state"=w6434, "Acquisition in"=w6435) -> ("error out"=w6421:errorcluster, "Acquisition out"=w6422:refnum<class "Acquisition.lvclass">)  [unwired: 7 in]
            n2646 = call-dynamic "Read Channel.vi"("error in (no error)"=w6421, "Acquisition in"=w6422) -> ("error out"=w6428:errorcluster, "Channel.lvclass"=w6424:refnum<class "Channel.lvclass">, "Acquisition out"=w6425:refnum<class "Acquisition.lvclass">)  [unwired: 7 in]
            n2647 = call "Read connected.vi"("error in (no error)"=w6428, "Device in"=w6424) -> ("error out"=w6427:errorcluster, "connected"=w6426:bool, "Device out"=w6429:refnum<class "Channel.lvclass">)  [unwired: 7 in]
            n2648 = case shown="True" w6426 {
              tunnel: w6429 -> [w6438 w6448]
              tunnel: [w6438 w6446] -> w6423
              tunnel: w6427 -> [w6437 w6443]
              tunnel: [w6437 w6441] -> w6430
              frame False {
              }
              frame True {
                n2649 = call-dynamic "Read State Machine.vi"("error in (no error)"=w6443, "Device in"=w6448) -> ("error out"=w6439:errorcluster, "State Machine.lvclass"=w6440:refnum<class "State Machine.lvclass">, "Device out"=w6447:refnum<class "Channel.lvclass">)  [unwired: 7 in]
                n2650 = call "Next State.vi"("error in (no error)"=w6439, "New_State"=96, "State Machine in"=w6440) -> ("error out"=w6442:errorcluster, "State Machine out"=w6445:refnum<class "State Machine.lvclass">)  [unwired: 7 in]
                n2651 = call-dynamic "Write State Machine.vi"("error in (no error)"=w6442, "State Machine.lvclass"=w6445, "Device in"=w6447) -> ("error out"=w6441:errorcluster, "Device out"=w6446:refnum<class "Channel.lvclass">)  [unwired: 7 in]
              }
            }
            n2652 = call-dynamic "Write Channel.vi"("error in (no error)"=w6430, "Channel.lvclass"=w6423, "Acquisition in"=w6425) -> ("error out"=w6420:errorcluster, "Acquisition out"=w6419:refnum<class "Acquisition.lvclass">)  [unwired: 7 in]
          }
          frame True {
            # "obs type"
            # "suffix"
            # "object"
            n2653 = call "Read Instrument.lvclass.vi"("S4ACS_GUI in"=w6456) -> ("error out"=w6458:errorcluster, "Instrument.lvclass"=w6460:refnum<class "Instrument.lvclass">, "S4ACS_GUI out"=w6455:refnum<class "S4GUI.lvclass">)  [unwired: 8 in]
            n2654 = call "Read WPROT.vi"("error in (no error)"=w6458, "Instrument in"=w6460) -> ("error out"=w6457:errorcluster, "Opt_Selector.lvclass"=w6459:refnum<class "Opt_Selector.lvclass">)  [unwired: 7 in, 1 out]
            n2655 = call-dynamic "Read sequencia.vi"("error in (no error)"=w6457, "Opt_Selector in"=w6459) -> ("sequencia"=w6454:u16)  [unwired: 7 in, 2 out]
            n2656 = case shown="False" w6462 {
              tunnel: [0 w6519] -> w6461
              tunnel: w6454 -> [_ w6518]
              frame False {
                # "OV 20230424: \n#SEQ agora armazena as\nposições da lâmina utilizadas.\nNa fotometria, #SEQ=0"
                # "fotometria:"
              }
              frame True {
                # "OV 20230424: \n#SEQ agora armazena as\nposições da lâmina utilizadas.\nNa polarimetria, #SEQ=WPROT.sequencia"
                # "polarimetria:"
                n2657 = To Unsigned Long Integer(number=w6518) -> (unsigned 32bit integer=w6519:u32)
              }
            }
            n2658 = call-dynamic "Write Acq_state.vi"("error in (no error)"=w6485, "Acq_state"=u32 251, "Acquisition in"=w6490) -> ("error out"=w6491:errorcluster, "Acquisition out"=w6492:refnum<class "Acquisition.lvclass">)  [unwired: 7 in]
            n2659 = call-dynamic "Read Channel.vi"("error in (no error)"=w6491, "Acquisition in"=w6492) -> ("error out"=w6494:errorcluster, "Channel.lvclass"=w6495:refnum<class "Channel.lvclass">, "Acquisition out"=w6503:refnum<class "Acquisition.lvclass">)  [unwired: 7 in]
            n2660 = property on="Start ch4" class="Bool"(error in=w6485, "DisabledEnum"=T7."Disabled and Grayed Out" ("Disabled")) -> ()  [unwired: 1 in, 2 out]
            n2661 = call-dynamic "Read Interface.vi"("error in (no error)"=w6494, "Channel in"=w6495) -> ("error out"=w6515:errorcluster, "Interface.lvclass"=w6516:refnum<class "Interface.lvclass">, "Channel out"=w6514:refnum<class "Channel.lvclass">)  [unwired: 7 in]
            n2662 = call "Write Exposure Time.vi"("error in (no error)"=w6515, "Exposure Time"="Exptime ch4", "Interface in"=w6516) -> ("error out"=w6450:errorcluster, "Interface out"=w6453:refnum<class "Interface.lvclass">)  [unwired: 7 in]
            n2663 = call-dynamic "Write prev ExpTime.vi"("error in (no error)"=w6450, "prev ExpTime"="Exptime ch4", "Interface in"=w6453) -> ("error out"=w6451:errorcluster, "Interface out"=w6452:refnum<class "Interface.lvclass">)  [unwired: 7 in]
            n2664 = call-dynamic "Write # Index.vi"("error in (no error)"=w6451, "# Index"="Index ch4", "Interface in"=w6452) -> ("error out"=w6512:errorcluster, "Interface out"=w6513:refnum<class "Interface.lvclass">)  [unwired: 7 in]
            n2665 = call-dynamic "Write Suffix.vi"("error in (no error)"=w6512, "Suffix"=w6487, "Interface in"=w6513) -> ("error out"=w6511:errorcluster, "Interface out"=w6510:refnum<class "Interface.lvclass">)  [unwired: 7 in]
            n2666 = call-dynamic "Write ObsType.vi"("error in (no error)"=w6511, "ObsType"=w6481, "Interface in"=w6510) -> ("error out"=w6508:errorcluster, "Interface out"=w6509:refnum<class "Interface.lvclass">)  [unwired: 7 in]
            n2667 = call-dynamic "Write Object.vi"("error in (no error)"=w6508, "Object"=w6480, "Interface in"=w6509) -> ("error out"=w6507:errorcluster, "Interface out"=w6506:refnum<class "Interface.lvclass">)  [unwired: 7 in]
            n2668 = call-dynamic "Write Comments.vi"("error in (no error)"=w6507, "Comments"=w6486, "Interface in"=w6506) -> ("error out"=w6504:errorcluster, "Interface out"=w6505:refnum<class "Interface.lvclass">)  [unwired: 7 in]
            n2669 = call-dynamic "Write DS9.vi"("error in (no error)"=w6504, "DS9"="F", "Interface in"=w6505) -> ("error out"=w6477:errorcluster, "Interface out"=w6479:refnum<class "Interface.lvclass">)  [unwired: 7 in]
            n2670 = call-dynamic "Write Observer.vi"("error in (no error)"=w6477, "Observer"=w6475, "Interface in"=w6479) -> ("error out"=w6476:errorcluster, "Interface out"=w6478:refnum<class "Interface.lvclass">)  [unwired: 7 in]
            n2671 = call-dynamic "Write # Images.vi"("error in (no error)"=w6476, "# Images"="Exp ch4", "Interface in"=w6478) -> ("error out"=w6482:errorcluster, "Interface out"=w6483:refnum<class "Interface.lvclass">)  [unwired: 7 in]
            n2672 = property on="Exposure Time ch4" class="Slide (strict)"("Scale.Maximum"="Exptime ch4", "Scale.Minimum"=0.0 ("Scale.Range:Minimum")) -> ()  [unwired: 2 in, 2 out]
            n2673 = property on="Exposure Done ch4" class="Slide (strict)"("Scale.Maximum"="Exp ch4", "Scale.Minimum"=0.0 ("Scale.Range:Minimum")) -> ()  [unwired: 2 in, 2 out]
            n2674 = call-dynamic "Write Interface.vi"("error in (no error)"=w6482, "Interface.lvclass"=w6483, "Channel in"=w6514) -> ("error out"=w6496:errorcluster, "Channel out"=w6497:refnum<class "Channel.lvclass">)  [unwired: 7 in]
            n2675 = property on="Cycles Done ch4" class="Slide (strict)"("Scale.Maximum"="#cycles ch4", "Scale.Minimum"=0.0 ("Scale.Range:Minimum")) -> ()  [unwired: 2 in, 2 out]
            n2676 = call-dynamic "Write ciclos.vi"("error in (no error)"=w6496, "ciclos"="#cycles ch4", "Channel in"=w6497) -> ("error out"=w6473:errorcluster, "Channel out"=w6474:refnum<class "Channel.lvclass">)  [unwired: 7 in]
            n2677 = call-dynamic "Write sequencias.vi"("error in (no error)"=w6473, "sequencias"=w6461, "Channel in"=w6474) -> ("error out"=w6472:errorcluster, "Channel out"=w6471:refnum<class "Channel.lvclass">)  [unwired: 7 in]
            n2678 = call-dynamic "Write Channel.vi"("error in (no error)"=w6472, "Channel.lvclass"=w6471, "Acquisition in"=w6503) -> ("error out"=w6465:errorcluster, "Acquisition out"=w6489:refnum<class "Acquisition.lvclass">)  [unwired: 7 in]
            n2679 = call-dynamic "Write sequencias.vi"("error in (no error)"=w6465, "sequencias"=w6461, "S4GUI in"=w6455) -> ("error out"=w6468:errorcluster, "S4GUI out"=w6467:refnum<class "S4GUI.lvclass">)  [unwired: 7 in]
            n2680 = call-dynamic "Write ciclos.vi"("error in (no error)"=w6468, "ciclos"="#cycles ch4", "S4ACS_GUI in"=w6467) -> ("error out"=w6469:errorcluster, "S4ACS_GUI out"=w6470:refnum<class "S4GUI.lvclass">)  [unwired: 7 in]
            n2681 = call-dynamic "Write TotalCiclos.vi"("error in (no error)"=w6469, "TotalCiclos"="#cycles ch4", "S4GUI in"=w6470) -> ("error out"=w6464:errorcluster, "S4GUI out"=w6466:refnum<class "S4GUI.lvclass">)  [unwired: 7 in]
          }
        }
        n2682 = call-dynamic "Write AcquisitionD.vi"("error in (no error)"=w6395, "Acquisition.lvclass"=w6410, "S4ACS_GUI in"=w6394) -> ("error out"=w6409:errorcluster, "S4ACS_GUI out"=w6406:refnum<class "S4GUI.lvclass">)  [unwired: 7 in]
      }
      event "Exptime ch1": Value Change {
        n2683 = event-data() -> ("NewVal"=w6524:dbl)  [unwired: 1 in]
        n2684 = call-dynamic "Read AcquisitionA.vi"("error in (no error)"=w6523, "S4ACS_GUI in"=w6522) -> ("error out"=w6538:errorcluster, "Acquisition.lvclass"=w6539:refnum<class "Acquisition.lvclass">, "S4ACS_GUI out"=w6536:refnum<class "S4GUI.lvclass">)  [unwired: 7 in]
        n2685 = call-dynamic "Read Channel.vi"("error in (no error)"=w6538, "Acquisition in"=w6539) -> ("error out"=w6527:errorcluster, "Channel.lvclass"=w6528:refnum<class "Channel.lvclass">, "Acquisition out"=w6529:refnum<class "Acquisition.lvclass">)  [unwired: 7 in]
        n2686 = call-dynamic "Read Interface.vi"("error in (no error)"=w6527, "Channel in"=w6528) -> ("error out"=w6533:errorcluster, "Interface.lvclass"=w6534:refnum<class "Interface.lvclass">, "Channel out"=w6532:refnum<class "Channel.lvclass">)  [unwired: 7 in]
        n2687 = call "Write Exposure Time.vi"("error in (no error)"=w6533, "Exposure Time"=w6524, "Interface in"=w6534) -> ("error out"=w6525:errorcluster, "Interface out"=w6526:refnum<class "Interface.lvclass">)  [unwired: 7 in]
        n2688 = call-dynamic "Write Interface.vi"("error in (no error)"=w6525, "Interface.lvclass"=w6526, "Channel in"=w6532) -> ("error out"=w6531:errorcluster, "Channel out"=w6530:refnum<class "Channel.lvclass">)  [unwired: 7 in]
        n2689 = call-dynamic "Write Channel.vi"("error in (no error)"=w6531, "Channel.lvclass"=w6530, "Acquisition in"=w6529) -> ("error out"=w6535:errorcluster, "Acquisition out"=w6537:refnum<class "Acquisition.lvclass">)  [unwired: 7 in]
        n2690 = call-dynamic "Write AcquisitionA.vi"("error in (no error)"=w6535, "Acquisition.lvclass"=w6537, "S4ACS_GUI in"=w6536) -> ("error out"=w6521:errorcluster, "S4ACS_GUI out"=w6520:refnum<class "S4GUI.lvclass">)  [unwired: 7 in]
      }
      event "Exp ch1": Value Change {
        n2691 = event-data() -> ("NewVal"=w6544:u32)  [unwired: 1 in]
        n2692 = call-dynamic "Read AcquisitionA.vi"("error in (no error)"=w6543, "S4ACS_GUI in"=w6542) -> ("error out"=w6558:errorcluster, "Acquisition.lvclass"=w6559:refnum<class "Acquisition.lvclass">, "S4ACS_GUI out"=w6556:refnum<class "S4GUI.lvclass">)  [unwired: 7 in]
        n2693 = call-dynamic "Read Channel.vi"("error in (no error)"=w6558, "Acquisition in"=w6559) -> ("error out"=w6547:errorcluster, "Channel.lvclass"=w6548:refnum<class "Channel.lvclass">, "Acquisition out"=w6549:refnum<class "Acquisition.lvclass">)  [unwired: 7 in]
        n2694 = call-dynamic "Read Interface.vi"("error in (no error)"=w6547, "Channel in"=w6548) -> ("error out"=w6553:errorcluster, "Interface.lvclass"=w6554:refnum<class "Interface.lvclass">, "Channel out"=w6552:refnum<class "Channel.lvclass">)  [unwired: 7 in]
